vi "2400-read(VISA).vi"(5 "2400 VISA ID":refnum<visa-resource-name>="GPIB0::24::INSTR") -> (0 "Voltage":dbl format="%.3e", 1 "Current":dbl format="%.4e", 2 "Time":dbl format="%.2e", 3 "Parameter3":dbl format="%.3e", 4 "Parameter5":dbl format="%.3e", 6 "String Output (Voltage, Current":string)   [LabVIEW 2018]
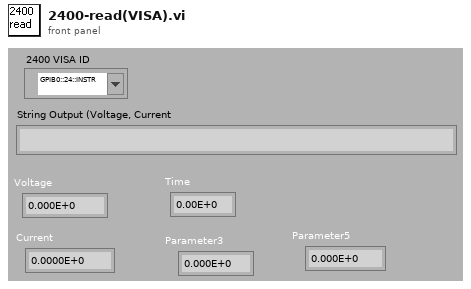
[diagram p1: front panel]
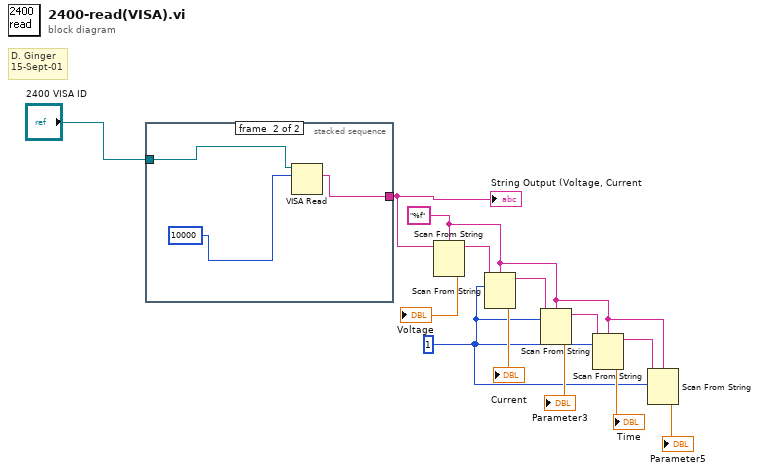
[diagram p0: block diagram]
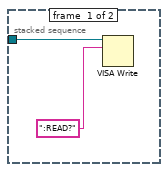
[diagram p2: hidden frame]
diagram:
  w2 = 1
  w4 = "%f" ("Format String")
  # "D. Ginger\n15-Sept-01"
  n1 = stacked-sequence {
    tunnel: [_ w16] -> w13
    tunnel: "2400 VISA ID" -> [w14 w17]
    frame #0 {
      n2 = VISA Write(VISA resource name=w14, write buffer=":READ?") -> ()  [unwired: 1 in, 3 out]
    }
    frame #1 {
      n3 = VISA Read(VISA resource name=w17, byte count=10000) -> (read buffer=w16:string)  [unwired: 1 in, 3 out]
    }
  }
  "String Output (Voltage, Current" <- w13
  n4 = Scan From String(format string=w4, input string=w13) -> (remaining string=w10:string, output 1=→"Voltage":dbl)  [unwired: 2 in, 3 out]
  n5 = Scan From String(format string=w4, input string=w10, initial scan location=w2) -> (remaining string=w12:string, output 1=→"Current":dbl)  [unwired: 1 in, 3 out]
  n6 = Scan From String(format string=w4, input string=w12, initial scan location=w2) -> (remaining string=w11:string, output 1=→"Parameter3":dbl)  [unwired: 1 in, 3 out]
  n7 = Scan From String(format string=w4, input string=w11, initial scan location=w2) -> (remaining string=w5:string, output 1=→"Time":dbl)  [unwired: 1 in, 3 out]
  n8 = Scan From String(format string=w4, input string=w5, initial scan location=w2) -> (output 1=→"Parameter5":dbl)  [unwired: 1 in, 4 out]
